vi "Test 2 button dialog.vi"() -> ()   [LabVIEW 2010]
uses:
  _TypeDefs/OK Button_TouchScreen.ctl
panel:
  in  "T button name (\"OK\")":string="If you know the pixel width and height of an image, this section will calculate the physical size (in inches) of the image when it is printed or displayed on various devices.\nTo use the calculator, enter the width and height, then select the output resolution which will be used.\n\n* Most monitors display images at approximately 75DPI. To check your own monitor, use the chart below.\n\n** Many printers use a process known as Image Refinement when processing images. This may impact the relation between input and output resolution. Generally, 300DPI is adequate for photo-like prints."
  out "T button?":T1
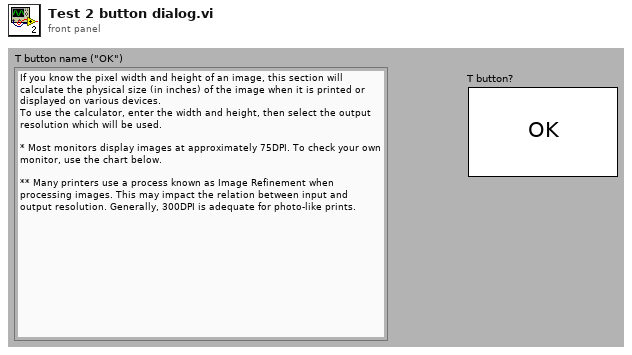
[diagram p1: front panel]
types:
  T1 = typedef "OK Button_TouchScreen.ctl" = bool
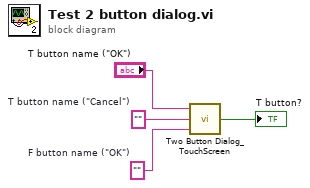
[diagram p0: block diagram]
diagram:
  w2 = ""  # T button name ("Cancel")
  w1 = ""  # F button name ("OK")
  n1 = call "Two Button Dialog_TouchScreen.vi"("F button name (\"Cancel\")"=w1, "T button name (\"OK\")"=w2, "Message"="T button name (\"OK\")") -> ("T Button?"=→"T button?":T1)
